vi "config_subVI.vi"() -> (0 "B out":dbl, 1 "A out":dbl, 2 "error out":errorcluster, 3 "task out":refnum<k21>)   [LabVIEW 2020]
uses:
  <vilib>/DAQmx/create/channels.llb/DAQmx Create Channel (AI-Voltage-Basic).vi
panel:
  in  "stop":bool
  in  "B":dbl
  in  "A":dbl
  in  "Physical Channel":tag
  # "y=Ax+B"
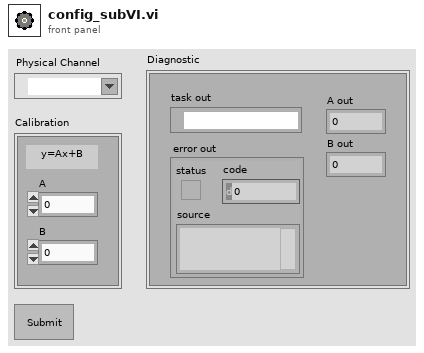
[diagram p1: front panel]
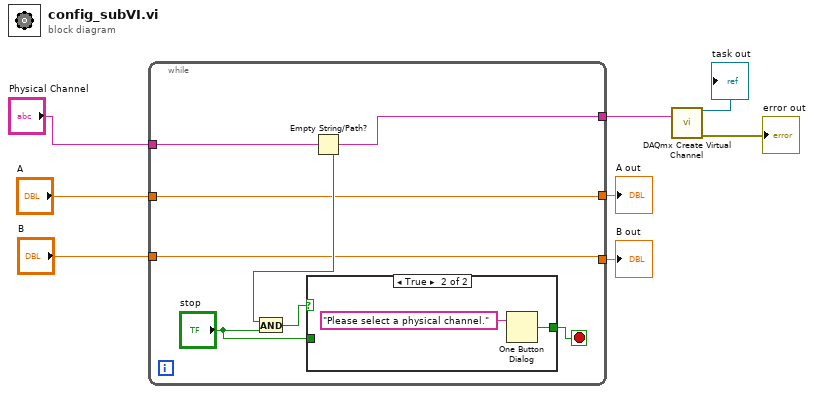
[diagram p0: block diagram]
diagram:
  n1 = while {
    tunnel: [w10] -> w5
    tunnel: [w9] -> w4
    tunnel: [w11] -> w6
    tunnel: "Physical Channel" -> [w11]
    tunnel: "A" -> [w10]
    tunnel: "B" -> [w9]
    stop <- w13 stop-if-true
    n2 = Empty String/Path?(string/path=w11) -> (empty?=w15:bool)
    n3 = And(x=w15, y="stop") -> (x .and. y?=w14:bool)
    n4 = case shown="True" w14 {
      tunnel: [w16 w17] -> w13
      tunnel: "stop" -> [w16 _]
      frame False {
      }
      frame True {
        n5 = One Button Dialog(message="Please select a physical channel.") -> (true=w17:bool)  [unwired: 1 in]
      }
    }
  }
  "A out" <- w5
  "B out" <- w4
  n6 = call-poly <vilib>:"DAQmx Create Virtual Channel.vi"("physical channels"=w6) -> ("task out"=→"task out":refnum<k21>, "error out"=→"error out":errorcluster)  [unwired: 13 in]
